vi "Remote Panel Multiple Server.vi"() -> ()   [LabVIEW 2024]
doc: "This Server VI serves as a model of how you could allow a client to only run a VI once after connecting and taking control. It starts the remote panel server, polls for a connection, waits until the client runs the VI once, and then locks control and disconnects the client."
uses:
  Remote Panels Globals.vi
panel:
  in  "Limit Connections":i32=1 caption="Limit Conn."
  out "Status":string[][](table)
  out "Active":bool
  in  "stop":bool
  out "Remote Panel Server Address":string
  out "Port":u16
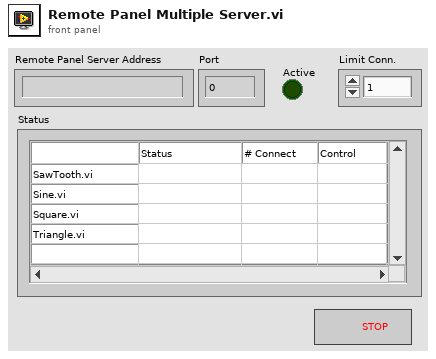
[diagram p1: front panel]
types:
  T1 = enum32{"Bad", "Idle", "Run top level", "Running"}
  T2 = typedef "LVRemotePanelConnectionsTypeDef.ctl" = cluster{"VI Name":string, "Remote":string, "UserName":string, "Port":i32, "Status":enum32{"Viewing", "Waiting For Control", "Controlling"}, "Create Time":timestamp, "Status Time":timestamp, "Control End Time":timestamp}[]
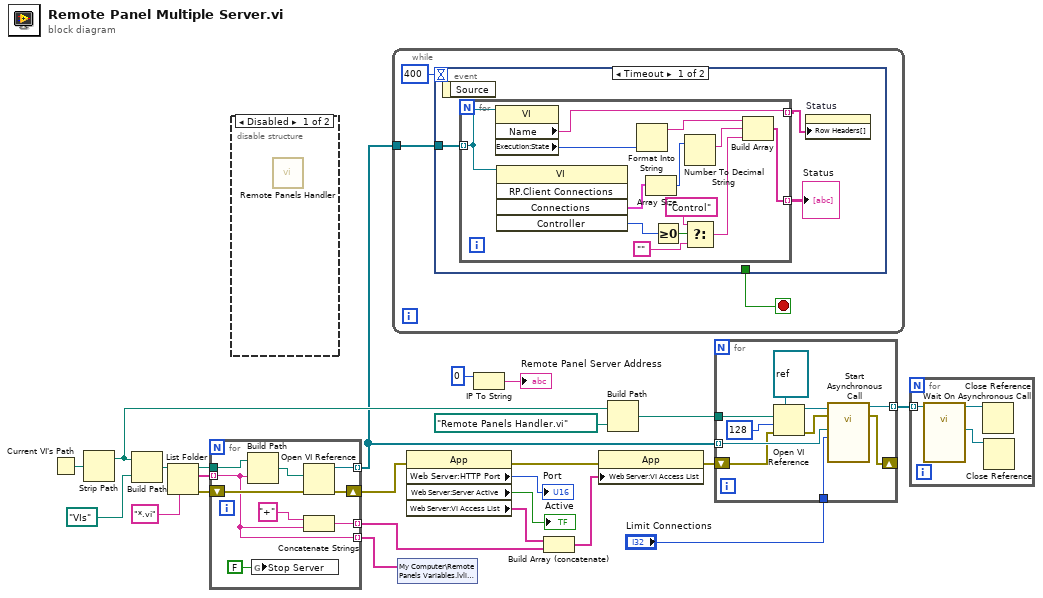
[diagram p0: block diagram]
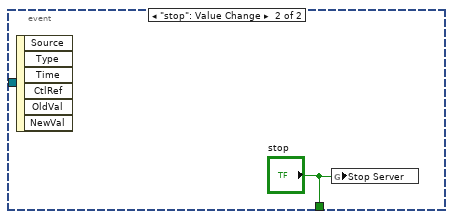
[diagram p2: hidden frame]
diagram:
  n1 = Current VI's Path() -> (path=w6:path)
  n2 = Strip Path(path=w6) -> (stripped path=w10:path)  [unwired: 1 out]
  n3 = Build Path(base path=w10, name or relative path=path "VIs") -> (appended path=w17:path)
  n4 = List Folder(path=w17, pattern="*.vi") -> (path out=w14:path, filenames=w15:string[], error out=w12:errorcluster)  [unwired: 2 in, 1 out]
  n5 = for {
    tunnel: w15 -> [w25] mode=indexing
    tunnel: w14 -> [w33]
    tunnel: [w30] -> w3 mode=indexing
    tunnel: [w27] -> w5 mode=indexing
    shift-right: [w29] -> w13
    shift-left: w12 -> [w28]
    tunnel: [w25] -> w2 mode=indexing
    n6 = Build Path(base path=w33, name or relative path=w25) -> (appended path=w32:path)
    n7 = global write "Remote Panels Globals.vi" "Stop Server"(FALSE ("Stop Server")) -> ()
    n8 = Open VI Reference(vi path=w32, error in (no error)=w28) -> (vi reference=w27:refnum<vi>, error out=w29:errorcluster)  [unwired: 4 in]
    n9 = Concatenate Strings("+" ("string"), w25) -> (w30:string)
  }
  n10 = disable-structure shown="Disabled" {
    frame Disabled {
      n11 = call "Remote Panels Handler.vi"() -> ()  [unwired: 10 in, 2 out]
    }
    frame Enabled {
    }
  }
  n12 = while {
    tunnel: w5 -> [w34]
    stop <- w36 stop-if-true
    n13 = event shown="[0] Timeout" {
      selector: _ -> [_ _]
      dyn-events: _ -> [_ _]
      timeout: 400 -> [_ _]
      tunnel: [_ "stop"] -> w36
      tunnel: w34 -> [w39 _]
      event Timeout {
        n14 = event-data() -> ()  [unwired: 1 in, 1 out]
        n15 = for {
          tunnel: w39 -> [w52] mode=indexing
          tunnel: [w41] -> w38 mode=indexing
          tunnel: [w40] -> w37 mode=indexing
          n16 = property class="VI"(reference=w52) -> ("Name"=w40:string, "Execution:State"=w51:T1)  [unwired: 1 in, 2 out]
          n17 = invoke class="VI" method="RP.Client Connections"(reference=w52) -> ("Connections"=w47:T2, "Controller"=w46:i32)  [unwired: 4 in, 3 out]
          n18 = Format Into String(w51) -> (resulting string=w50:string)  [unwired: 3 in, 1 out]
          n19 = Array Size(array=w47) -> (size(s)=w49:i32)
          n20 = Greater Or Equal To 0?(x=w46) -> (x >= 0?=w45:bool)
          n21 = Number To Decimal String(number=w49) -> (decimal integer string=w48:string)  [unwired: 1 in]
          n22 = Select(t="Control", s=w45, f="") -> (s? t:f=w42:string)
          n23 = Build Array(w50, w48, w42) -> (w41:string[])
        }
        "Status" <- w38
        n24 = property on="Status" class="Tbl (strict)"("Row Headers[]"=w37) -> ()  [unwired: 2 in, 2 out]
      }
      event "stop": Value Change {
        n25 = event-data() -> ()  [unwired: 1 in, 6 out]
        n26 = global write "Remote Panels Globals.vi" "Stop Server"("stop") -> ()
      }
    }
  }
  n27 = shared-variable "My Computer\\Remote Panels Variables.lvlib\\VIsList"(w2) -> ()  [unwired: 1 in, 1 out]
  n28 = property class="App"(error in=w13) -> (error out=w21:errorcluster, "Web Server:HTTP Port"=→"Port":u16, "Web Server:Server Active"=→"Active":bool, "Web Server:VI Access List"=w23:string[])  [unwired: 1 in, 1 out]
  n29 = IP To String(2:u32 0 ("net address")) -> (0:→"Remote Panel Server Address":string)  [unwired: 1 in]
  n30 = Build Array (concatenate)(w23, w3) -> (w22:string[])
  n31 = property class="App"(error in=w21, "Web Server:VI Access List"=w22) -> (error out=w7:errorcluster)  [unwired: 1 in, 1 out]
  n32 = Build Path(base path=w10, name or relative path=path "Remote Panels Handler.vi") -> (appended path=w9:path)
  n33 = for {
    tunnel: w5 -> [w58] mode=indexing
    tunnel: w9 -> [w63]
    tunnel: [w59] -> w8 mode=indexing
    shift-right: [w55] -> _
    shift-left: w7 -> [w57]
    tunnel: "Limit Connections" -> [w54]
    n34 = Open VI Reference(type specifier VI Refnum (for type only)=refnum<vi> refnum, vi path=w63, options=128, error in (no error)=w57) -> (vi reference=w60:refnum<vi>, error out=w56:errorcluster)  [unwired: 2 in]
    n35 = call-by-ref "Start Asynchronous Call"(reference=w60, error in=w56, "Limit  connections"=w54, "VI in"=w58) -> (reference out=w59:refnum<vi>, error out=w55:errorcluster)  [unwired: 8 in, 2 out]
  }
  n36 = for {
    tunnel: w8 -> [w66] mode=indexing
    n37 = call-by-ref "Wait On Asynchronous Call"(reference=w66) -> (reference out=w65:refnum<vi>, "VI out"=w64:refnum<vi>)  [unwired: 11 in, 2 out]
    n38 = Close Reference(reference=w65) -> ()  [unwired: 1 in, 1 out]
    n39 = Close Reference(reference=w64) -> ()  [unwired: 1 in, 1 out]
  }
